vi "SetGetSyncClass.vi"(7 "Set? (f)":bool, 11 "SyncPluginBase in":refnum<class "SyncPluginBase.lvclass">) -> (3 "SyncPluginBase out":refnum<class "SyncPluginBase.lvclass">)   [LabVIEW 2014, in "SyncPlugins.lvlib" / "SyncPluginBase.lvclass"]
uses:
  SyncPluginBase.lvclass
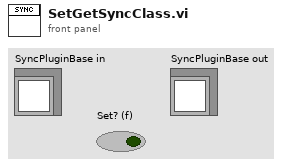
[diagram p1: front panel]
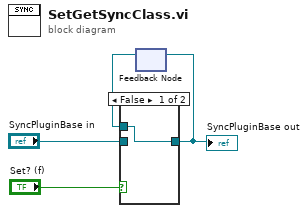
[diagram p0: block diagram]
diagram:
  n1 = feedback #1() -> (w1:refnum<class "SyncPluginBase.lvclass">)  [unwired: 1 in]
  n2 = case shown="False" "Set? (f)" {
    tunnel: "SyncPluginBase in" -> [_ w6]
    tunnel: [w5 w6] -> w2
    tunnel: w1 -> [w5 _]
    frame False {
    }
    frame True {
    }
  }
  "SyncPluginBase out" <- w2
  n3 = feedback-in #1(w2) -> ()
